vi "Begin.vi"() -> (1 "Темп-ра":dbl, 2 "№ об-ца":dbl, 3 "String":string)   [LabVIEW 2018]
panel:
  in  "№ образца:":dbl
  in  "Температура:":dbl
  in  "ОК (ОЗ)":bool
  in  "ОА(ОП)":bool
  out "Лампа":bool=TRUE
  # "Тип индикатора:"
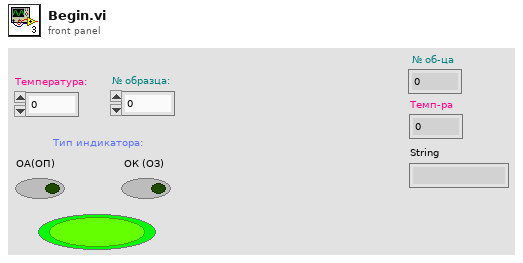
[diagram p1: front panel]
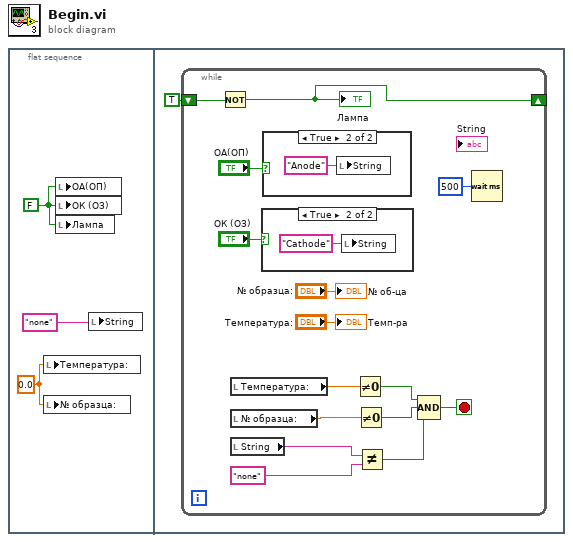
[diagram p0: block diagram]
diagram:
  n1 = flat-sequence {
    frame #0 {
      w1 = 0.0 ("Температура:")
      w3 = FALSE ("ОА (ОП)")
      n2 = local write "Температура:"(w1) -> ()
      n3 = local write "№ образца:"(w1) -> ()
      n4 = local write "ОА(ОП)"(w3) -> ()
      n5 = local write "ОК (ОЗ)"(w3) -> ()
      n6 = local write "Лампа"(w3) -> ()
      n7 = local write "String"("none" ("String")) -> ()
    }
    frame #1 {
      n8 = while {
        shift-right: [w17] -> _
        shift-left: TRUE -> [w18]
        stop <- w9 stop-if-true
        n9 = Not(x=w18) -> (.not. x?=w17:bool)
        "Лампа" <- w17
        n10 = local read "Температура:"() -> (w6:dbl)
        n11 = local read "№ образца:"() -> (w5:dbl)
        n12 = local read "String"() -> (w16:string)
        n13 = case shown="True" "ОК (ОЗ)" {
          frame False {
          }
          frame True {
            n14 = local write "String"("Cathode" ("String")) -> ()
          }
        }
        n15 = case shown="True" "ОА(ОП)" {
          frame False {
          }
          frame True {
            n16 = local write "String"("Anode" ("String")) -> ()
          }
        }
        n17 = Not Equal To 0?(x=w6) -> (x != 0?=w12:bool)
        n18 = Not Equal To 0?(x=w5) -> (x != 0?=w11:bool)
        n19 = Not Equal?(x=w16, y="none") -> (x != y?=w10:bool)
        n20 = Compound Arithmetic op=AND(w12, w11, w10) -> (w9:bool)
        n21 = Wait (ms)(milliseconds to wait=u32 500) -> ()  [unwired: 1 out]
        "№ об-ца" <- "№ образца:"
        "Темп-ра" <- "Температура:"
      }
    }
  }
